vi "UpdateCounterCfg.vi"(10 "name":string, 11 "Variant":variant) -> ()   [LabVIEW 2017, in "NEVSTOP QD Shortcuts.lvlib"]
uses:
  NEVSTOP QD Shortcuts.lvlib
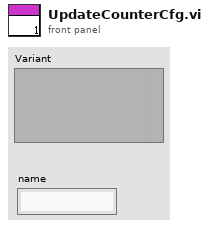
[diagram p1: front panel]
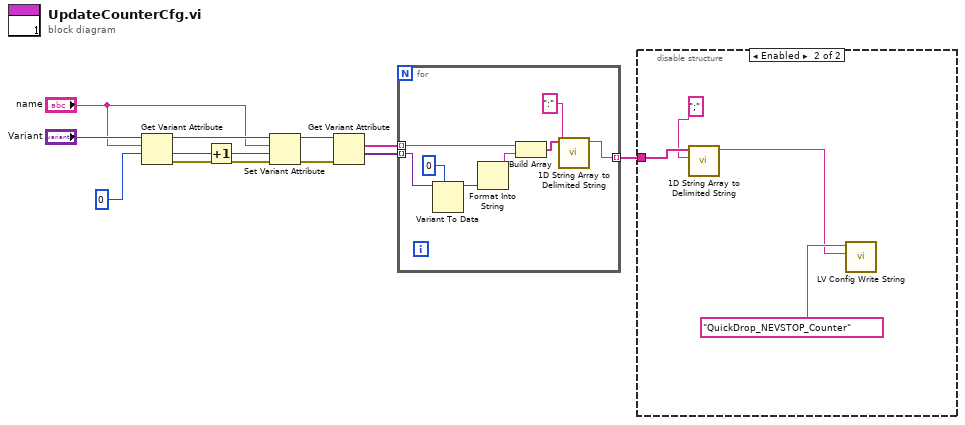
[diagram p0: block diagram]
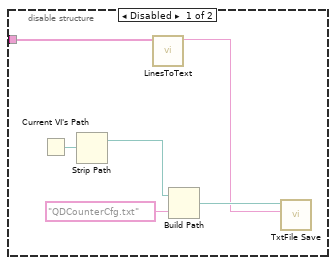
[diagram p2: hidden frame]
diagram:
  n1 = Get Variant Attribute(Variant="Variant", name="name", default value (empty Variant)=0) -> (duplicate Variant=w7:variant, value=w3:i32, error out=w6:errorcluster)  [unwired: 1 in, 1 out]
  n2 = Increment(x=w3) -> (x+1=w1:i32)
  n3 = Set Variant Attribute(Variant=w7, name="name", value=w1, error in=w6) -> (Variant out=w5:variant, error out=w4:errorcluster)  [unwired: 1 out]
  n4 = Get Variant Attribute(Variant=w5, error in=w4) -> (names=w11:string[], values=w12:variant[])  [unwired: 2 in, 2 out]
  n5 = for {
    tunnel: w12 -> [w18] mode=indexing
    tunnel: w11 -> [w20] mode=indexing
    tunnel: [w13] -> w10 mode=indexing
    n6 = Variant To Data(type=0, Variant=w18) -> (data=w17:i32)  [unwired: 1 in, 1 out]
    n7 = Format Into String(w17) -> (resulting string=w19:string)  [unwired: 3 in, 1 out]
    n8 = Build Array(w20, w19) -> (w15:string[])
    n9 = call "1D String Array to Delimited String.vi"("delimiter"=":" ("delimiter (Tab)"), "string array"=w15) -> ("delimited string"=w13:string)  [unwired: 9 in]
  }
  n10 = disable-structure shown="Enabled" {
    disable-tunnel: w10 -> [w25 w30]
    frame Disabled {
      n11 = Current VI's Path() -> (path=w22:path)
      n12 = Strip Path(path=w22) -> (stripped path=w21:path)  [unwired: 1 out]
      n13 = call "LinesToText.vi"("Lines"=w25) -> ("string"=w23:string)  [unwired: 9 in, 1 out]
      n14 = Build Path(base path=w21, name or relative path="QDCounterCfg.txt") -> (appended path=w24:path)
      n15 = call "TxtFile Save.vi"("text"=w23, "Path"=w24) -> ()  [unwired: 9 in, 1 out]
    }
    frame Enabled {
      n16 = call "1D String Array to Delimited String.vi"("delimiter"=";" ("delimiter (Tab)"), "string array"=w30) -> ("delimited string"=w27:string)  [unwired: 9 in]
      n17 = call <resource>:"LV Config Write String.vi"("value"=w27, "key"="QuickDrop_NEVSTOP_Counter") -> ()  [unwired: 5 in, 1 out]
    }
  }
